vi "Update Logging Enabled Channel.vi"(6 "Trigger Event":refnum<user-event>, 7 "System Time":timestamp, 8 "error in (no error)":errorcluster, 10 "Command Values in":dbl[](array[numeric]), 11 "Log Info in":T1 {"Node ID" format="%.0x"; "TDMS Error Code"."Data Ref" format="%.0x"; "Missed Samples"."Data Ref" format="%.0x"; "File Status"."Data Ref" format="%.0x"; "Start New File"."Data Ref" format="%.0x"; "Logging Enabled"."Data Ref" format="%.0x"; "Stop Trigger"."Node Data Ref" format="%.0x"; "Stop Trigger"."Node ID" format="%.0x"; "Start Trigger"."Node Data Ref" format="%.0x"; "Start Trigger"."Node ID" format="%.0x"}) -> (0 "error out":errorcluster, 2 "Command Values out":dbl[](array[numeric]), 3 "Log Info out":T1 {"Node ID" format="%.0x"; "TDMS Error Code"."Data Ref" format="%.0x"; "Missed Samples"."Data Ref" format="%.0x"; "File Status"."Data Ref" format="%.0x"; "Start New File"."Data Ref" format="%.0x"; "Logging Enabled"."Data Ref" format="%.0x"; "Stop Trigger"."Node Data Ref" format="%.0x"; "Stop Trigger"."Node ID" format="%.0x"; "Start Trigger"."Node Data Ref" format="%.0x"; "Start Trigger"."Node ID" format="%.0x"})   [LabVIEW 2015, in "Waveform Data Logger Engine.lvlib"]
uses:
  Waveform Data Logger Engine.lvlib
  Types/Trigger Event Data.ctl
  Types/Trigger Received.ctl
  Types/Inline Waveform Log Info.ctl
  Classes/Log File Specifications/Waveform TDMS Log File Specification/Waveform TDMS Log File Specification.lvclass
  Classes/Triggers/Trigger/Trigger.lvclass
  <vilib>/NI Veristand/Custom Device API/Custom Device Item Ref.ctl
  Types/Inline Log Waveform.ctl
  Types/Trigger Settings.ctl
  Types/Log Status.ctl
  Types/Channel.ctl
  <vilib>/NI Veristand/Custom Device API/Data Reference.ctl
  Classes/Triggers/Trigger/Trigger.lvclass/Trigger.ctl
  Classes/Triggers/Digital Edge Trigger/Digital Edge Trigger.lvclass/Digital Edge Trigger.ctl
  Classes/Triggers/Analog Edge Trigger/Analog Edge Trigger.lvclass/Analog Edge Trigger.ctl
  Classes/Triggers/Value Change Trigger/Value Change Trigger.lvclass/Value Change Trigger.ctl
  Classes/Triggers/Trigger/Initialize.vi
  Classes/Triggers/Digital Edge Trigger/Initialize Digital Edge Trigger.vi
  Classes/Triggers/Analog Edge Trigger/Initialize Analog Edge Trigger.vi
  Classes/Triggers/Value Change Trigger/Initialize Value Change Trigger.vi
  Classes/Triggers/Value Change Trigger/Value Change Trigger.lvclass
  Classes/Triggers/Analog Edge Trigger/Analog Edge Trigger.lvclass
  Classes/Triggers/Digital Edge Trigger/Digital Edge Trigger.lvclass
  <vilib>/NI Veristand/Custom Device API/Custom Device API.lvlib
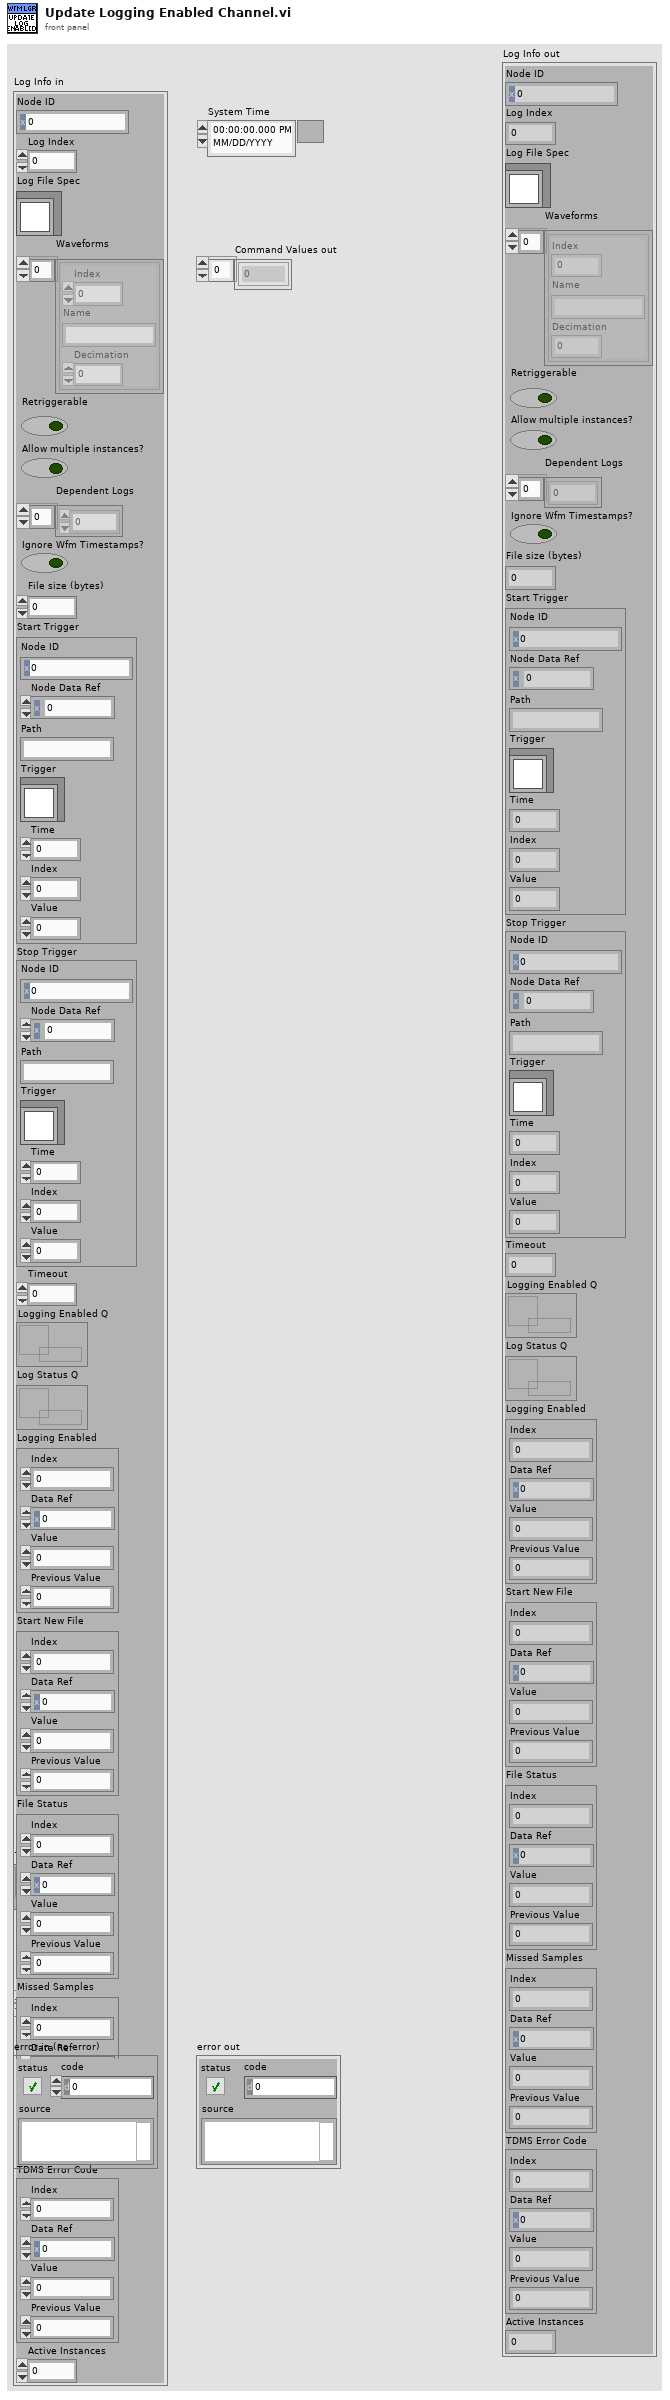
[diagram p1: front panel]
types:
  T1 = typedef "Waveform Data Logger Engine.lvlib/Inline Waveform Log Info.ctl" = cluster{"Node ID":T2, "Log Index":i32, "Log File Spec":refnum<class "Waveform TDMS Log File Specification.lvclass">, "Waveforms":T3[], "Retriggerable":bool, "Allow multiple instances?":bool, "Dependent Logs":i32[], "Ignore Wfm Timestamps?":bool, "File size (bytes)":i64, "Start Trigger":T4, "Stop Trigger":T4, "Timeout":dbl, "Logging Enabled Q":refnum<queue>, "Log Status Q":refnum<queue>, "Logging Enabled":T5, "Start New File":T5, "File Status":T5, "Missed Samples":T5, "TDMS Error Code":T5, "Active Instances":i32}
  T2 = typedef "Custom Device API.lvlib/Custom Device Item Ref.ctl" = u64
  T3 = typedef "Waveform Data Logger Engine.lvlib/Inline Log Waveform.ctl" = cluster{"Index":i32, "Name":string, "Decimation":u32}
  T4 = typedef "Waveform Data Logger Engine.lvlib/Trigger Settings.ctl" = cluster{"Node ID":T2, "Node Data Ref":i32, "Path":string, "Trigger":refnum<class "Trigger.lvclass">, "Time":dbl, "Index":i32, "Value":dbl}
  T5 = typedef "Waveform Data Logger Engine.lvlib/Channel.ctl" = cluster{"Index":i32, "Data Ref":T6, "Value":dbl, "Previous Value":dbl}
  T6 = typedef "Custom Device API.lvlib/Data Reference.ctl" = i32
  T7 = typedef "Waveform Data Logger Engine.lvlib/Trigger Received.ctl" = enum16{"None", "Start", "Stop", "Both", "Disable"}
  T8 = typedef "Waveform Data Logger Engine.lvlib/Trigger Event Data.ctl" = cluster{"Log Index":i32, "Trigger Received":T7, "Start Trigger Time":timestamp, "Stop Trigger Time":timestamp}
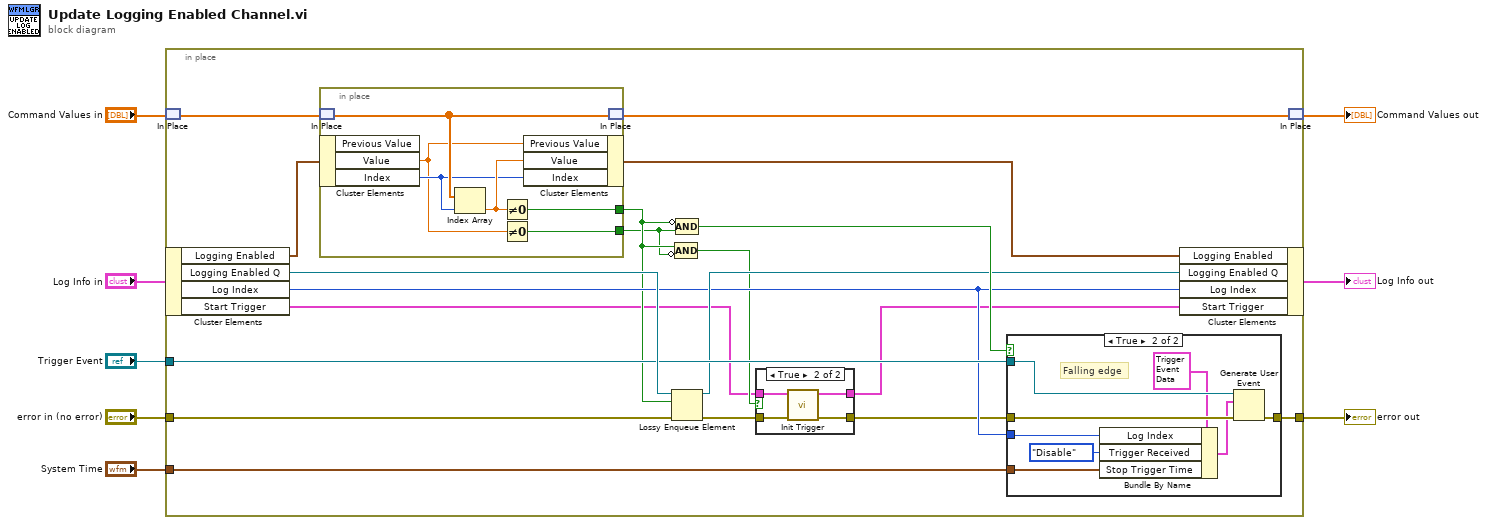
[diagram p0: block diagram]
diagram:
  n1 = in-place {
    in-place-border: "error in (no error)" -> [w26]
    in-place-border: [w21] -> w7
    in-place-border: "Trigger Event" -> [w22]
    in-place-border: "System Time" -> [w18]
    n2 = in-place-match #1("Command Values in") -> (w17:dbl[])
    n3 = in-place-cluster #2("Log Info in") -> ("Logging Enabled"=w27:T5, "Logging Enabled Q"=w24:refnum<queue>, "Log Index"=w19:i32, "Start Trigger"=w11:T4)
    n4 = in-place {
      in-place-border: [w45] -> w15
      in-place-border: [w44] -> w14
      n5 = in-place-match #3(w17) -> (w48:dbl[])
      n6 = in-place-cluster #4(w27) -> ("Value"=w43:dbl, "Index"=w46:i32)  [unwired: 1 out]
      n7 = Index Array(array=w48, index=w46) -> (element=w47:dbl)
      n8 = Not Equal To 0?(x=w47) -> (x != 0?=w45:bool)
      n9 = Not Equal To 0?(x=w43) -> (x != 0?=w44:bool)
      n10 = in-place-cluster #4("Previous Value"=w43, "Value"=w47, "Index"=w46) -> (w25:T5)
      n11 = in-place-match #3(w48) -> (w16:dbl[])
    }
    n12 = Lossy Enqueue Element(queue=w24, element=w15, error in (no error)=w26) -> (queue out=w20:refnum<queue>, error out=w12:errorcluster)  [unwired: 2 out]
    n13 = Compound Arithmetic op=AND(w15, invert w14) -> (w13:bool)
    n14 = Compound Arithmetic op=AND(invert w15, w14) -> (w23:bool)
    n15 = case shown="True" w13 {
      tunnel: w12 -> [w29 w33]
      tunnel: w11 -> [w28 w31]
      tunnel: [w28 w30] -> w10
      tunnel: [w29 w32] -> w9
      frame False {
      }
      frame True {
        n16 = call "Init Trigger.vi"("error in (no error)"=w33, "Trigger in"=w31) -> ("error out"=w32:errorcluster, "Trigger out"=w30:T4)  [unwired: 8 in]
      }
    }
    n17 = case shown="True" w23 {
      tunnel: w9 -> [w34 w42]
      tunnel: w22 -> [_ w41]
      tunnel: [w34 w40] -> w21
      tunnel: w19 -> [_ w36]
      tunnel: w18 -> [_ w35]
      frame False {
      }
      frame True {
        # "Falling edge"
        n18 = Bundle By Name(cluster=T8 {"Log Index"=0, "Trigger Received"=enum."None", "Start Trigger Time"=timestamp(0 s since 1904-01-01), "Stop Trigger Time"=timestamp(0 s since 1904-01-01)} ("event data"), "Log Index"=w36, "Trigger Received"=Trigger_Received."Disable", "Stop Trigger Time"=w35) -> (w38:T8)
        n19 = Generate User Event(user event=w41, event data cluster=w38, error in=w42) -> (error out=w40:errorcluster)  [unwired: 1 in, 1 out]
      }
    }
    n20 = in-place-cluster #2("Logging Enabled"=w25, "Logging Enabled Q"=w20, "Log Index"=w19, "Start Trigger"=w10) -> (→"Log Info out":T1)
    n21 = in-place-match #1(w16) -> (→"Command Values out":dbl[])
  }
  "error out" <- w7
